vi "NT Get Persistence.vi"(8 "error in":errorcluster, 11 "Name":string="Numeric") -> (0 "error out":errorcluster, 3 "Persistence":bool=TRUE)   [LabVIEW 2017]
doc: "Write the double precision numeric to the named entry."
uses:
  <vilib>/Rock Robotics/Network Tables/Create Actual Table Name.vi
  <vilib>/Rock Robotics/Network Tables/Table Manager.vi
  <vilib>/Rock Robotics/Network Tables/NT Globals.vi
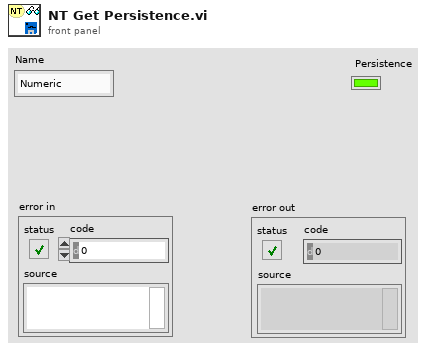
[diagram p1: front panel]
types:
  T1 = enum16{"Add", "Remove", "Clear", "Init", "Retrieve"}
  T2 = typedef "Field ID.ctl" = i32
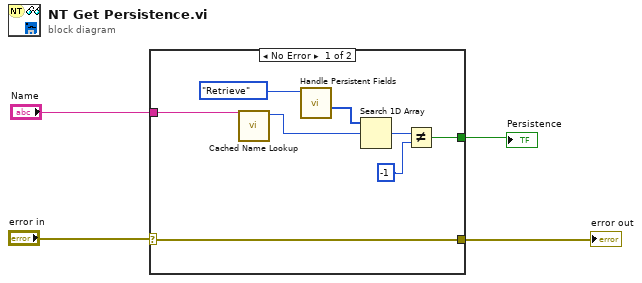
[diagram p0: block diagram]
diagram:
  n1 = case shown="No Error" "error in" {
    selector: "error in" -> [w12 w13]
    tunnel: "Name" -> [w11 _]
    tunnel: [w12 w13] -> w2
    tunnel: [w5 _] -> w1
    frame No Error {
      n2 = call <vilib>:"Cached Name Lookup.vi"("Name"=w11) -> ("Entry ID"=w8:T2)  [unwired: 8 in, 2 out]
      n3 = call <vilib>:"Handle Persistent Fields.vi"("Operation"=T1."Retrieve") -> ("Field IDs out"=w9:T2[])  [unwired: 10 in]
      n4 = Search 1D Array(1D array=w9, element=w8) -> (index of element=w7:i32)  [unwired: 1 in]
      n5 = Not Equal?(x=w7, y=-1) -> (x != y?=w5:bool)
    }
    frame Error {
    }
  }
  "error out" <- w2
  "Persistence" <- w1
